vi "Calculate Frequency factor.vi"(9 "TLcu":dbl=21.0 format="%#_12f", 10 "OkFreq":dbl=64.0 format="%0#_12f", 11 "MeasuredFreq":dbl=63.999367 format="%#_12f") -> (1 "Adj Factor":u8[](array[numeric]) format="%x", 2 "Adj Factor":string, 3 "PPM":dbl format="%#_13f")   [LabVIEW 2009]
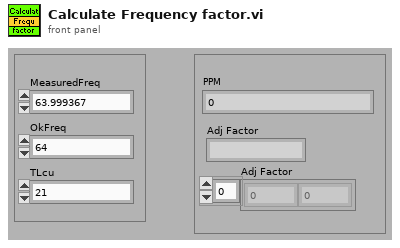
[diagram p1: front panel]
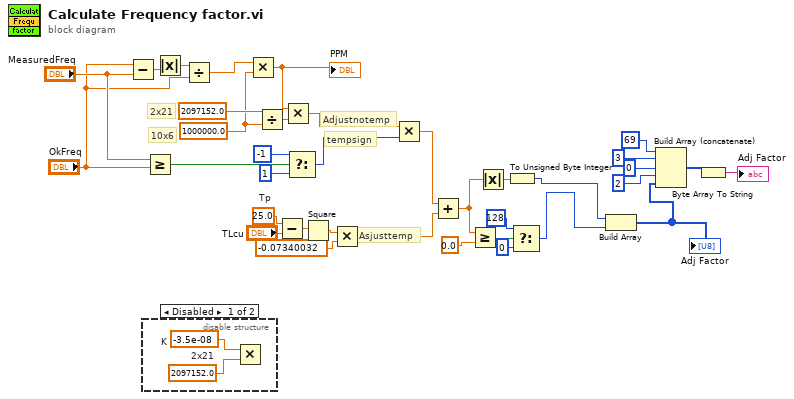
[diagram p0: block diagram]
diagram:
  w32 = 25.0  # Tp
  w12 = 1000000.0 ("y")
  # "tempsign"
  # "Adjustnotemp"
  # "Asjusttemp"
  # "10x6"
  # "2x21"
  n1 = Subtract(x="OkFreq", y="MeasuredFreq") -> (x-y=w20:dbl)
  n2 = disable-structure shown="Disabled" {
    frame #0 {
      w37 = 2097152.0  # 2x21
      w38 = -3.5e-08  # K
      n3 = Multiply(x=w38, y=w37) -> ()  [unwired: 1 out]
    }
    frame #1 {
    }
  }
  n4 = Greater Or Equal?(x="MeasuredFreq", y="OkFreq") -> (x >= y?=w26:bool)
  n5 = Absolute Value(x=w20) -> (abs(x)=w19:dbl)
  n6 = Divide(x=w19, y="OkFreq") -> (x/y=w11:dbl)
  n7 = Multiply(x=w11, y=w12) -> (x*y=w34:dbl)
  "PPM" <- w34
  n8 = Divide(x=2097152.0, y=w12) -> (x/y=w35:dbl)
  n9 = Subtract(x=w32, y="TLcu") -> (x-y=w31:dbl)
  n10 = Multiply(x=w34, y=w35) -> (x*y=w10:dbl)
  n11 = Select(t=i8 -1, s=w26, f=i8 1) -> (s? t:f=w23:i8)
  n12 = Square(x=w31) -> (x^2=w30:dbl)
  n13 = Multiply(x=w30, y=-0.07340032 ("x*y")) -> (x*y=w22:dbl)
  n14 = Multiply(x=w10, y=w23) -> (x*y=w21:dbl)
  n15 = Add(x=w21, y=w22) -> (x+y=w14:dbl)
  n16 = Greater Or Equal?(x=w14, y=0.0) -> (x >= y?=w15:bool)
  n17 = Absolute Value(x=w14) -> (abs(x)=w13:dbl)
  n18 = To Unsigned Byte Integer(number=w13) -> (unsigned 8bit integer=w3:u8)
  n19 = Select(t=u8 128, s=w15, f=u8 0) -> (s? t:f=w2:u8)
  n20 = Build Array(w3, w2) -> (w1:u8[])
  "Adj Factor" <- w1
  n21 = Build Array (concatenate)(u8 69 ("element"), u8 3 ("element"), u8 0 ("element"), u8 2 ("element"), w1) -> (w4:u8[])
  n22 = Byte Array To String(unsigned byte array=w4) -> (string=→"Adj Factor":string)
